vi "Remove Controls from Selection.vi"(8 "Error In":errorcluster, 11 "Selection":refnum<vi>[](array[refnum])) -> (0 "Error Out":errorcluster, 3 "Filtered Selection":refnum<vi>[](array[refnum]))   [LabVIEW 2017, in "Toolkit.lvlib"]
uses:
  Toolkit.lvlib
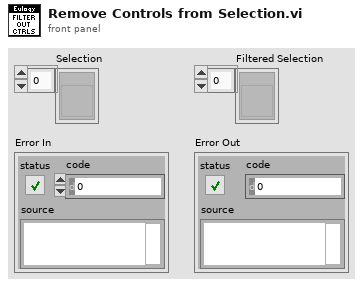
[diagram p1: front panel]
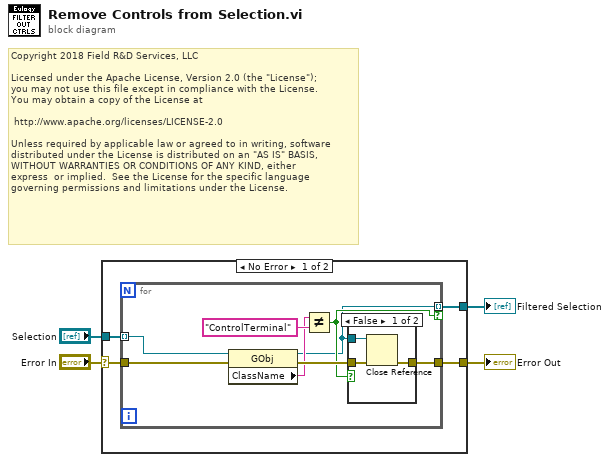
[diagram p0: block diagram]
diagram:
  # "Copyright 2018 Field R&D Services, LLC\n\nLicensed under the Apache License, Version 2.0 (the \"License\");\nyou may not use this file except in compliance with the License.\nYou may obtain a copy of the License at\n\n\thttp://www.apache.org/licenses/LICENSE-2.0\n\nUnless required by applicable law or agreed to in writing, software\ndistributed under the License is distributed on an \"AS IS\" BASIS,\nWITHOUT WARRANTIES OR CONDITIONS OF ANY KIND, either \nexpress  or implied.  See the License for the specific language \ngoverning permissions and limitations under the License."
  n1 = case shown="No Error" "Error In" {
    selector: "Error In" -> [w6 w21]
    tunnel: [w5 w22] -> w4
    tunnel: [w8 w21] -> w3
    tunnel: "Selection" -> [w7 w22]
    frame No Error {
      n2 = for {
        tunnel: w7 -> [w15] mode=indexing
        tunnel: [w9] -> w5 mode=indexing if=w10
        tunnel: w6 -> [w14]
        tunnel: [w11] -> w8
        n3 = property class="GObj"(reference=w15, error in=w14) -> (reference out=w9:refnum<vi>, error out=w13:errorcluster, "ClassName"=w12:string)
        n4 = Not Equal?(x=w12, y="ControlTerminal") -> (x != y?=w10:bool)
        n5 = case shown="False" w10 {
          tunnel: w13 -> [w19 w20]
          tunnel: [w18 w20] -> w11
          tunnel: w9 -> [w17 _]
          frame False {
            n6 = Close Reference(reference=w17, error in (no error)=w19) -> (error out=w18:errorcluster)
          }
          frame True {
          }
        }
      }
    }
    frame Error {
    }
  }
  "Filtered Selection" <- w4
  "Error Out" <- w3
